vi "SubVI.vi"(11 "dataflow in":bool) -> ()   [LabVIEW 2018]
uses:
  f272b586-ebd8-4b3c-9c37-11e2c20a5fda.vi
  f272b586-ebd8-4b3c-9c37-11e2c20a5fda.vi/caf2d4a3-5a7b-40e1-b7b0-74b52901b9f9.vi
  f272b586-ebd8-4b3c-9c37-11e2c20a5fda.vi/caf2d4a3-5a7b-40e1-b7b0-74b52901b9f9.vi/0a1ee2ab-da6d-4243-8cf3-8125e611a602.vi
  api/Log.vi
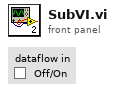
[diagram p1: front panel]
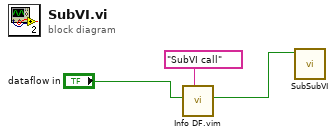
[diagram p0: block diagram]
diagram:
  n1 = call "Info DF.vim"("message"="SubVI call", "dataflow in"="dataflow in") -> ("dataflow out"=w3:bool)  [unwired: 9 in]
  n2 = call "SubSubVI.vi"("dataflow in"=w3) -> ()  [unwired: 11 in]
